vi "SumMatrix2Dto1D.vi"(10 "DIM":i32, 11 "M":dbl[][](array[numeric])) -> (3 "SUM(M,DIM)":dbl[](array[numeric]))   [LabVIEW 2014]
uses:
  <vilib>/Analysis/baseanly.llb/A x Vector.vi
  <vilib>/Analysis/NI_AALBase.lvlib
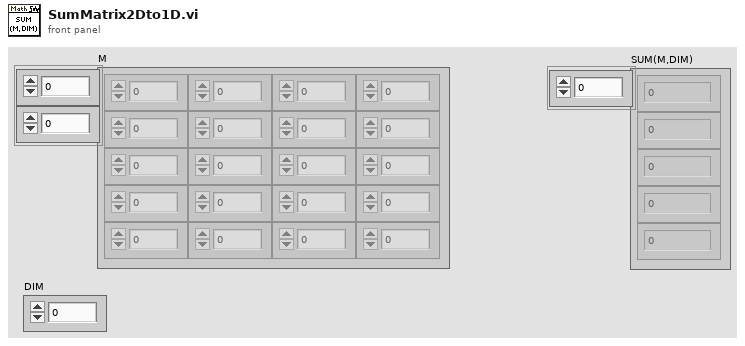
[diagram p1: front panel]
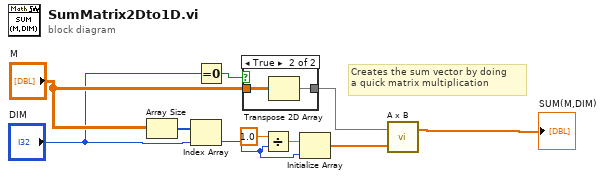
[diagram p0: block diagram]
diagram:
  # "Creates the sum vector by doing \na quick matrix multiplication"
  n1 = Array Size(array="M") -> (size(s)=w9:i32[])
  n2 = Index Array(array=w9, index="DIM") -> (element=w10:i32)
  n3 = Equal To 0?(x="DIM") -> (x = 0?=w2:bool)
  n4 = case shown="True" w2 {
    tunnel: "M" -> [w11 w13]
    tunnel: [w11 w12] -> w7
    frame False {
    }
    frame True {
      n5 = Transpose 2D Array(2D array=w13) -> (transposed array=w12:dbl[][])
    }
  }
  n6 = Divide(x=1.0, y=w10) -> (x/y=w4:dbl)
  n7 = Initialize Array(w4, w10) -> (w3:dbl[])
  n8 = call-poly <vilib>:"A x B.vi"("Vector"=w3, "A"=w7) -> ("A x Vector"=→"SUM(M,DIM)":dbl[])  [unwired: 1 out]
